vi "TestExec.Configure Select Master File Sync Config File.vi"(9 "Dialog":bool, 10 "File Sync Local":path, 11 "Working Config":path) -> (2 "Is Master":bool, 3 "File Sync File":path)   [LabVIEW 2018]
uses:
  <vilib>/Utility/config.llb/Read Key (String).vi
  <vilib>/Utility/config.llb/NI_LVConfig.lvlib
  <vilib>/KATE/Files/File Utils.lvlib
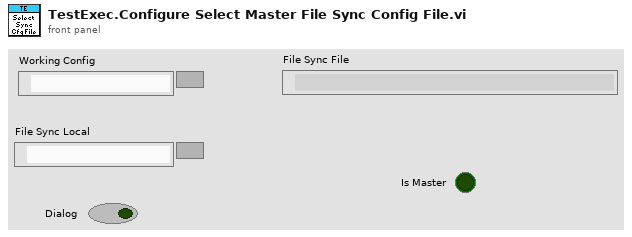
[diagram p1: front panel]
types:
  T1 = typedef "NI_LVConfig.lvlib/Config Data RefNum.ctl" = refnum<k1>
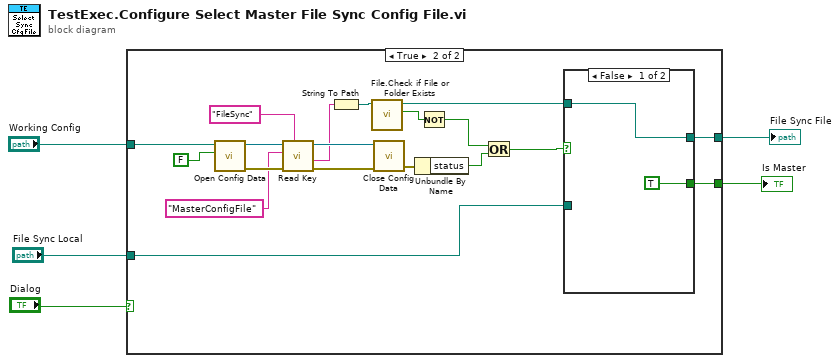
[diagram p0: block diagram]
diagram:
  n1 = case shown="True" "Dialog" {
    tunnel: "File Sync Local" -> [w6 w8]
    tunnel: [w6 w11] -> w3
    tunnel: "Working Config" -> [_ w23]
    tunnel: [_ w7] -> w1
    frame False {
    }
    frame True {
      n2 = call <vilib>:"Open Config Data.vi"("create file if necessary (T)"=FALSE, "configuration file path"=w23) -> ("error out"=w25:errorcluster, "refnum"=w24:T1)  [unwired: 7 in, 1 out]
      n3 = call-poly <vilib>:"Read Key.vi"("section"="FileSync", "error in (no error)"=w25, "key"="MasterConfigFile", "refnum"=w24) -> ("error out"=w18:errorcluster, "value"=w17:string, "refnum out"=w19:T1)  [unwired: 4 in, 1 out]
      n4 = String To Path(string=w17) -> (path=w16:path)
      n5 = call <vilib>:"File.Check if File or Folder Exists.vi"("Path"=w16) -> ("Exists"=w12:bool, "Dup Path"=w10:path)  [unwired: 6 in, 3 out]
      n6 = call <vilib>:"Close Config Data.vi"("error in (no error)"=w18, "refnum"=w19) -> ("error out"=w15:errorcluster)  [unwired: 8 in, 1 out]
      n7 = Unbundle By Name(w15) -> ("status"=w14:bool)
      n8 = Not(x=w12) -> (.not. x?=w13:bool)
      n9 = Or(x=w13, y=w14) -> (x .or. y?=w9:bool)
      n10 = case shown="False" w9 {
        tunnel: [w27 w28] -> w11
        tunnel: w10 -> [w27 _]
        tunnel: w8 -> [_ w28]
        tunnel: [TRUE _] -> w7
        frame False {
        }
        frame True {
        }
      }
    }
  }
  "File Sync File" <- w3
  "Is Master" <- w1
